vi "Test_CaseHandler.vi"(4 "data":string, 5 "action":string) -> (0 "error out":errorcluster, 1 "response":string)   [LabVIEW 2009]
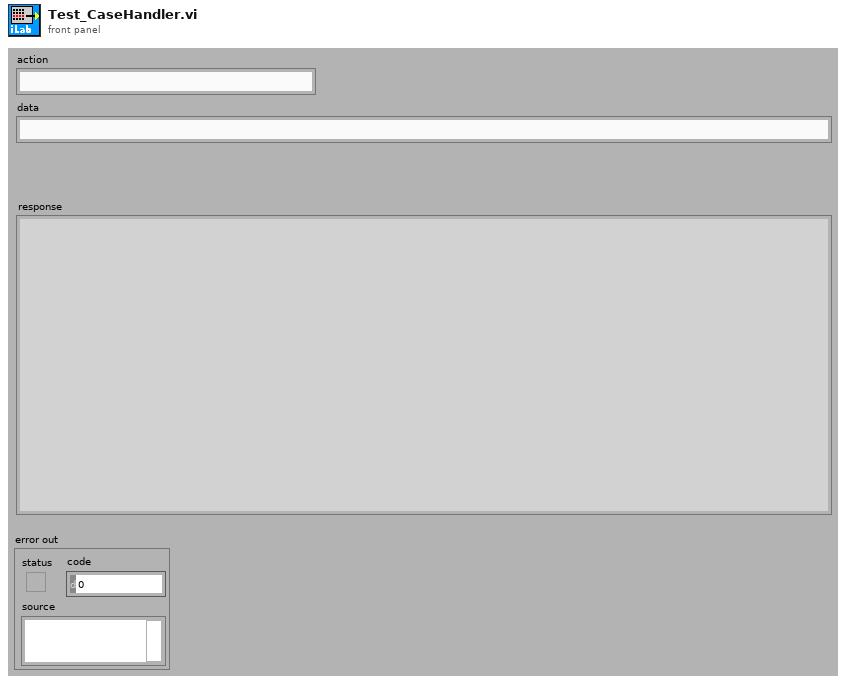
[diagram p1: front panel]
types:
  T1 = typedef "LVRemotePanelConnectionsTypeDef.ctl" = cluster{"VI Name":string, "Remote":string, "UserName":string, "Port":i32, "Status":enum32{"Viewing", "Waiting For Control", "Controlling"}, "Create Time":timestamp, "Status Time":timestamp, "Control End Time":timestamp}[]
  T2 = cluster{"VI Name":string, "Remote":string, "UserName":string, "Port":i32, "Status":enum32{"Viewing", "Waiting For Control", "Controlling"}, "Create Time":timestamp, "Status Time":timestamp, "Control End Time":timestamp}
  T3 = cluster{"Name":string, "Path":path, "Type String":string, "Display Name":string, "Type":string}
  T4 = enum32{"Bad", "Idle", "Run top level", "Running"}
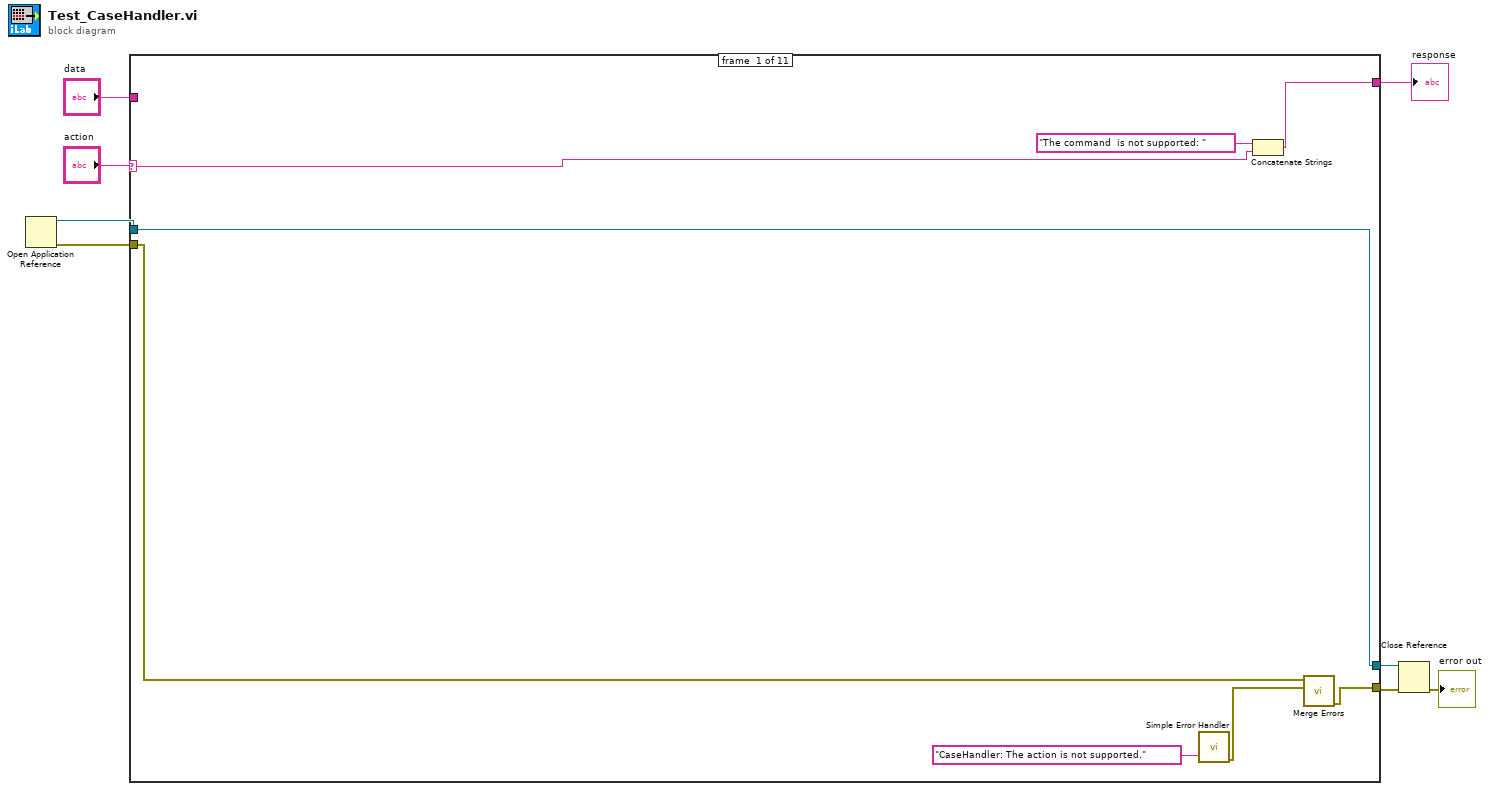
[diagram p0: block diagram]
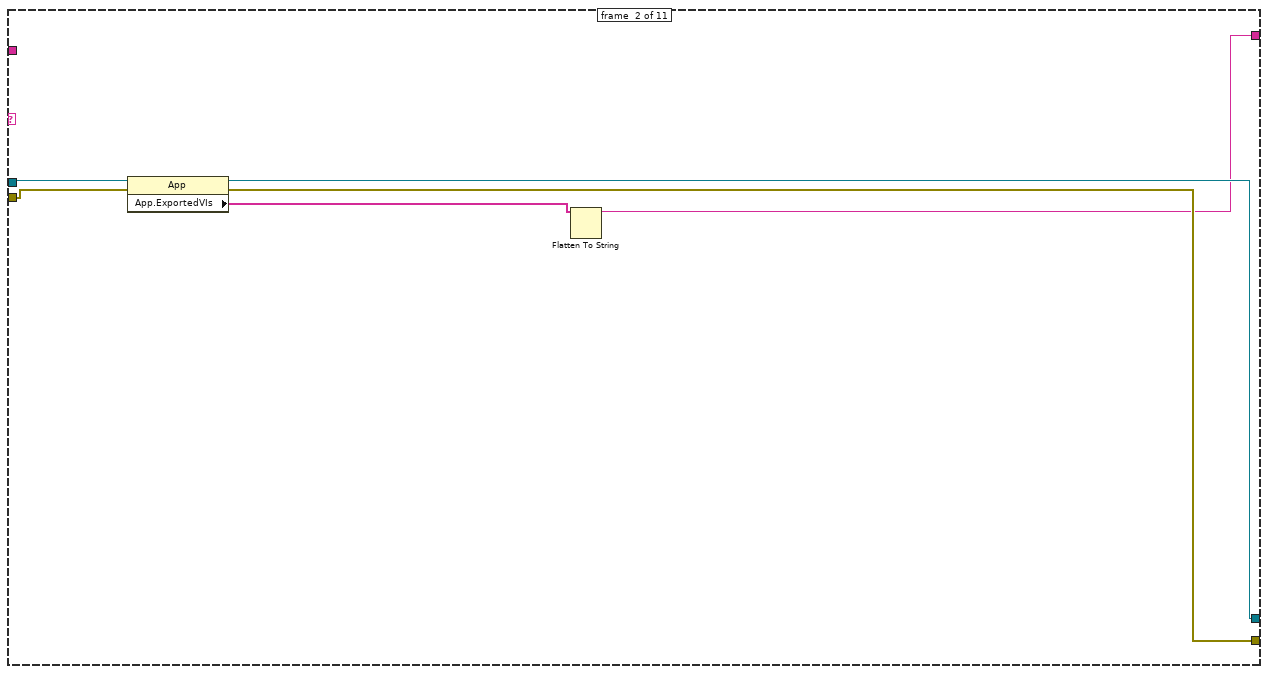
[diagram p2: hidden frame]
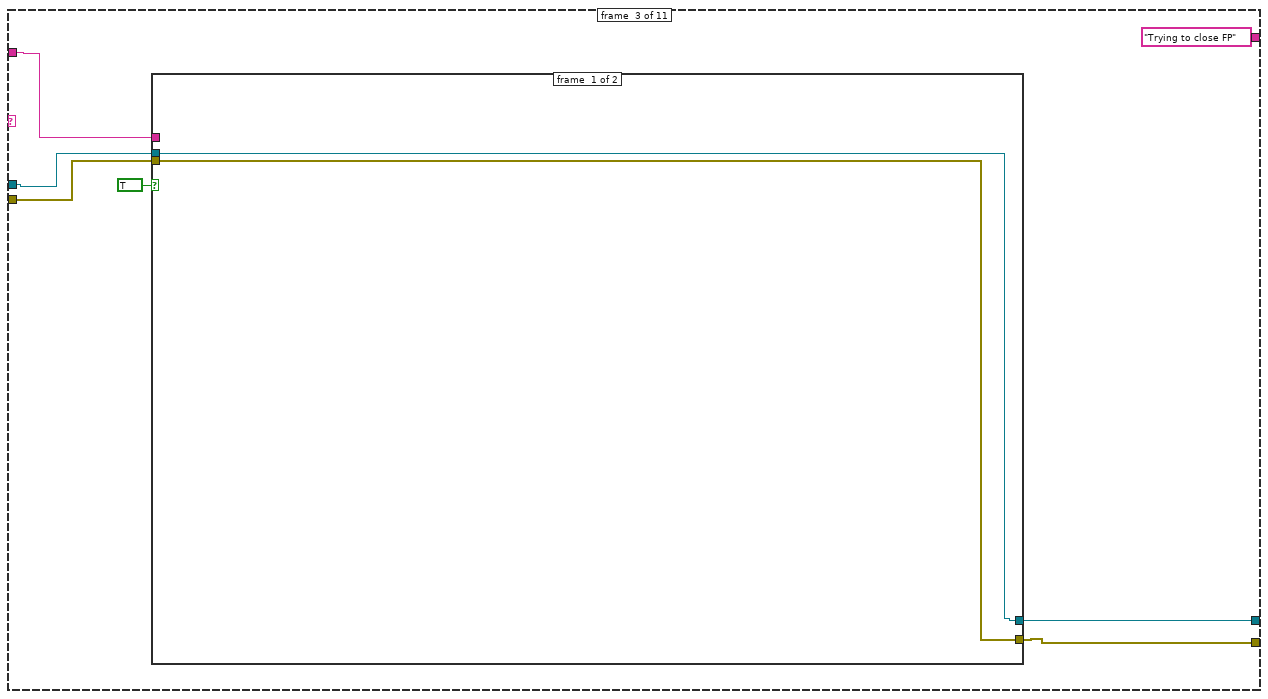
[diagram p3: hidden frame]
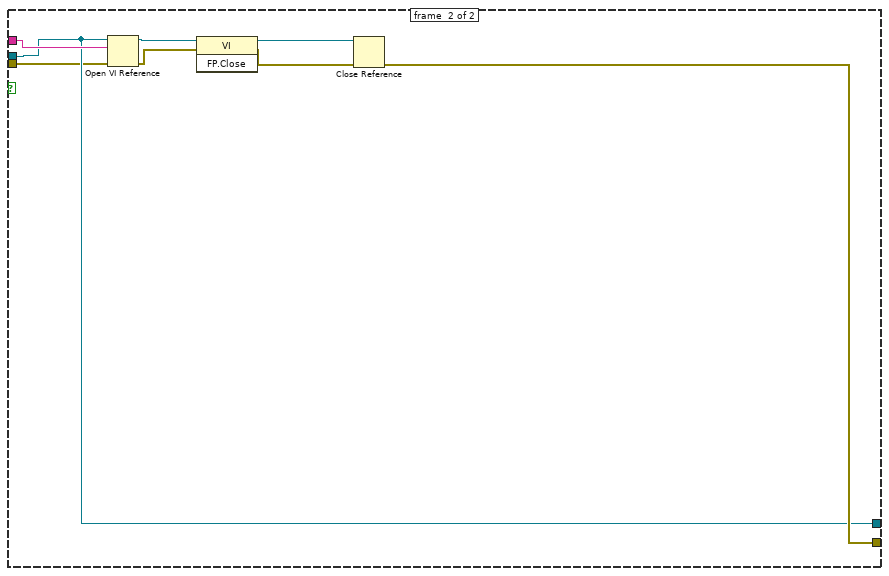
[diagram p4: hidden frame]
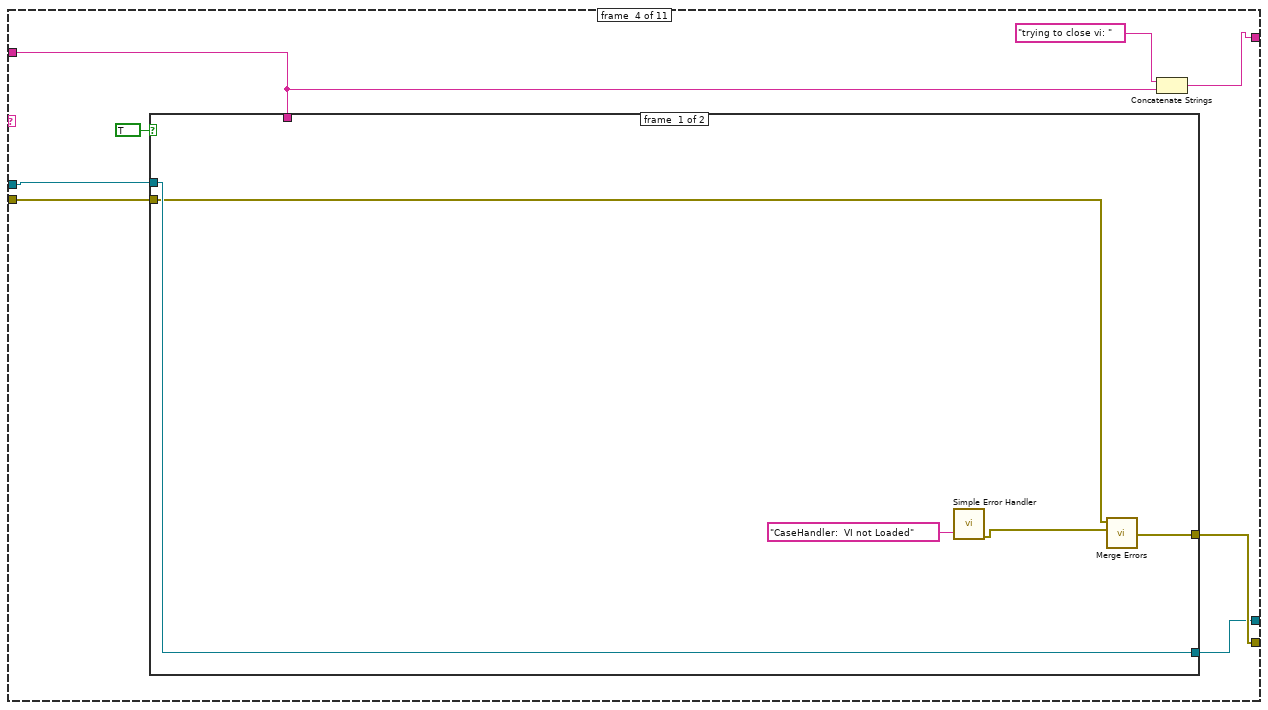
[diagram p5: hidden frame]
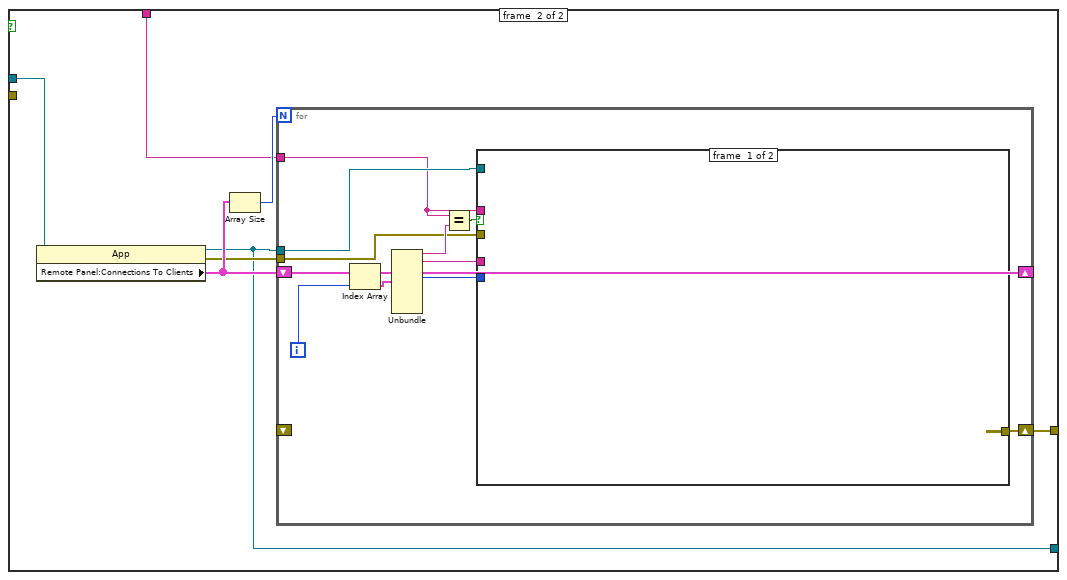
[diagram p6: hidden frame]
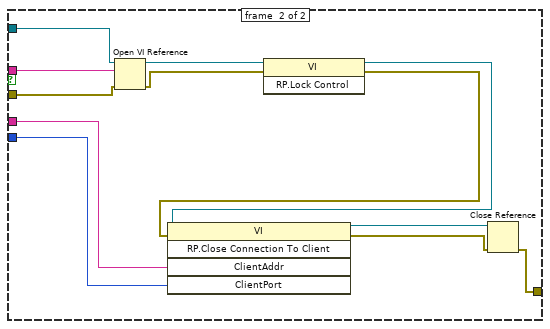
[diagram p7: hidden frame]
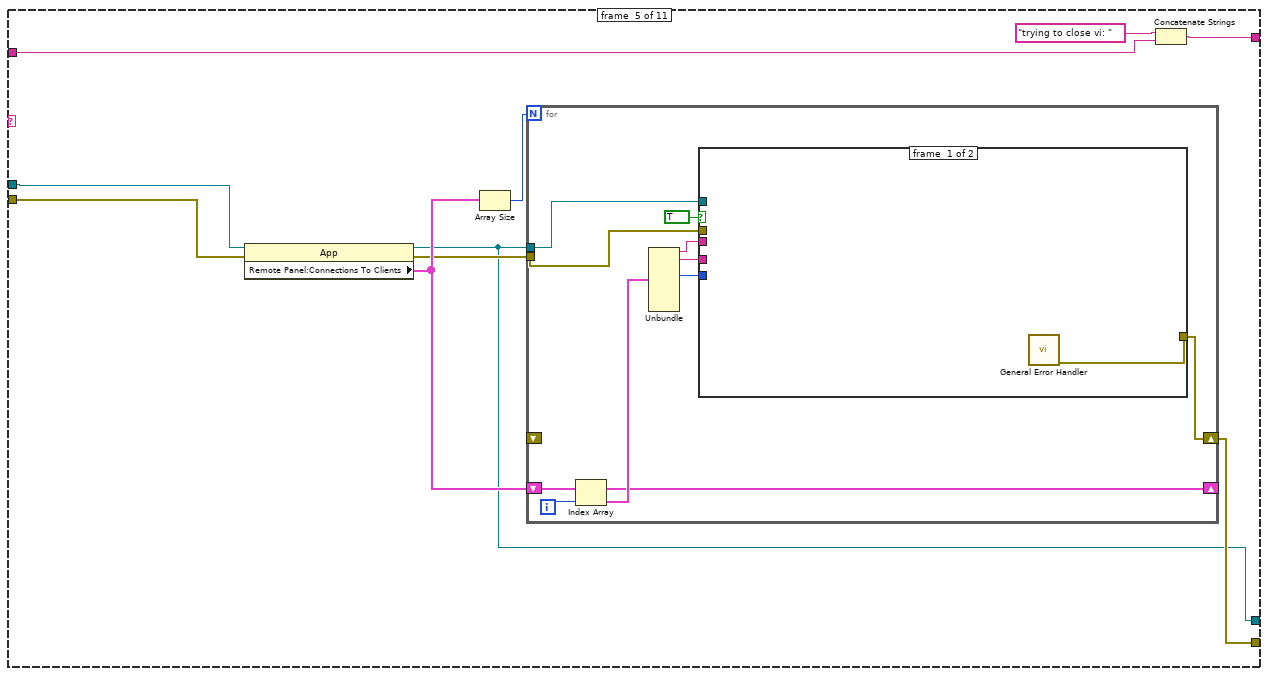
[diagram p8: hidden frame]
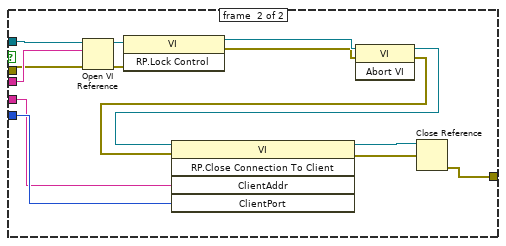
[diagram p9: hidden frame]
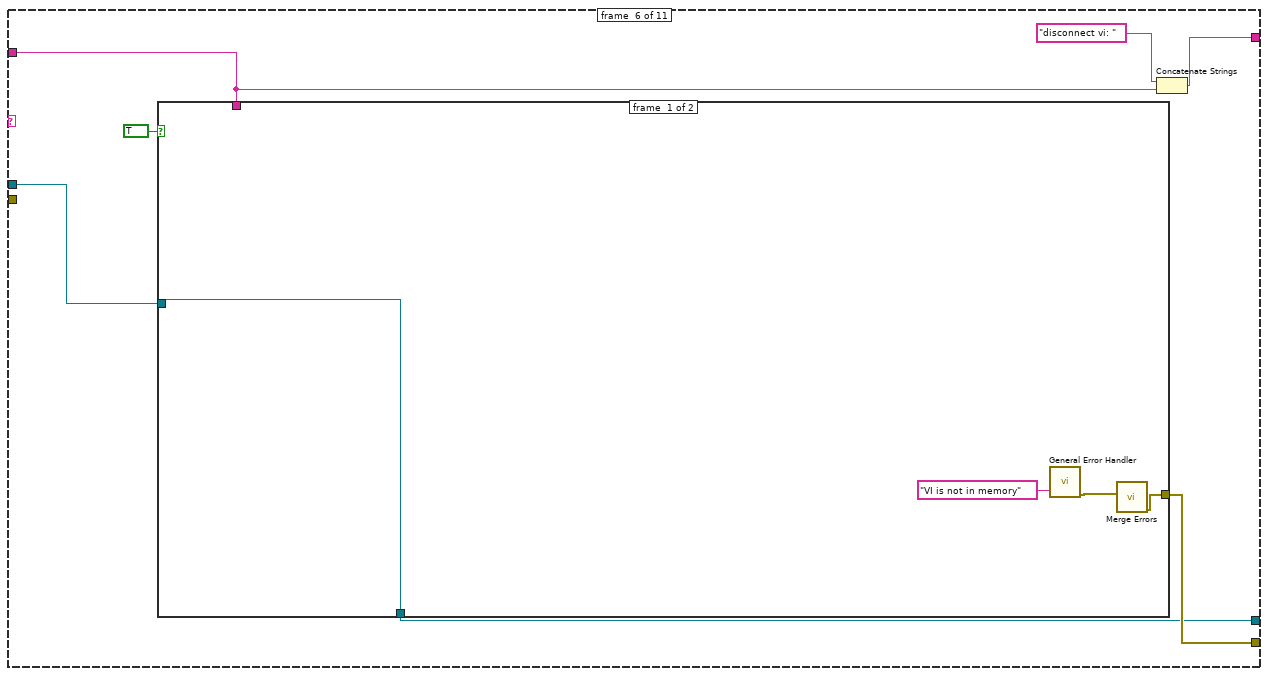
[diagram p10: hidden frame]
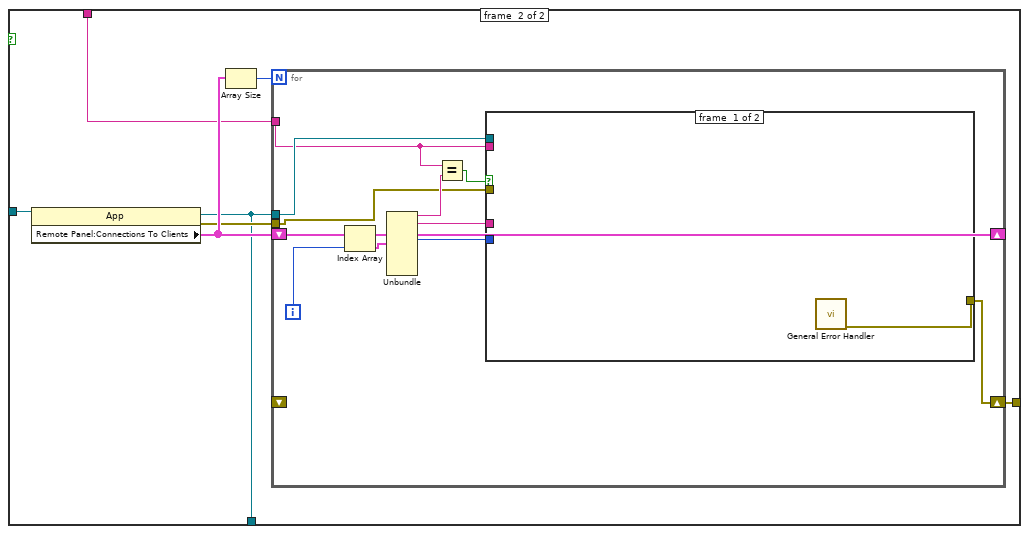
[diagram p11: hidden frame]
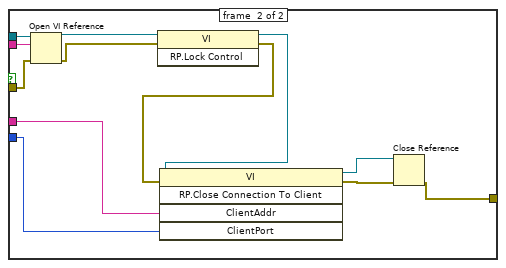
[diagram p12: hidden frame]
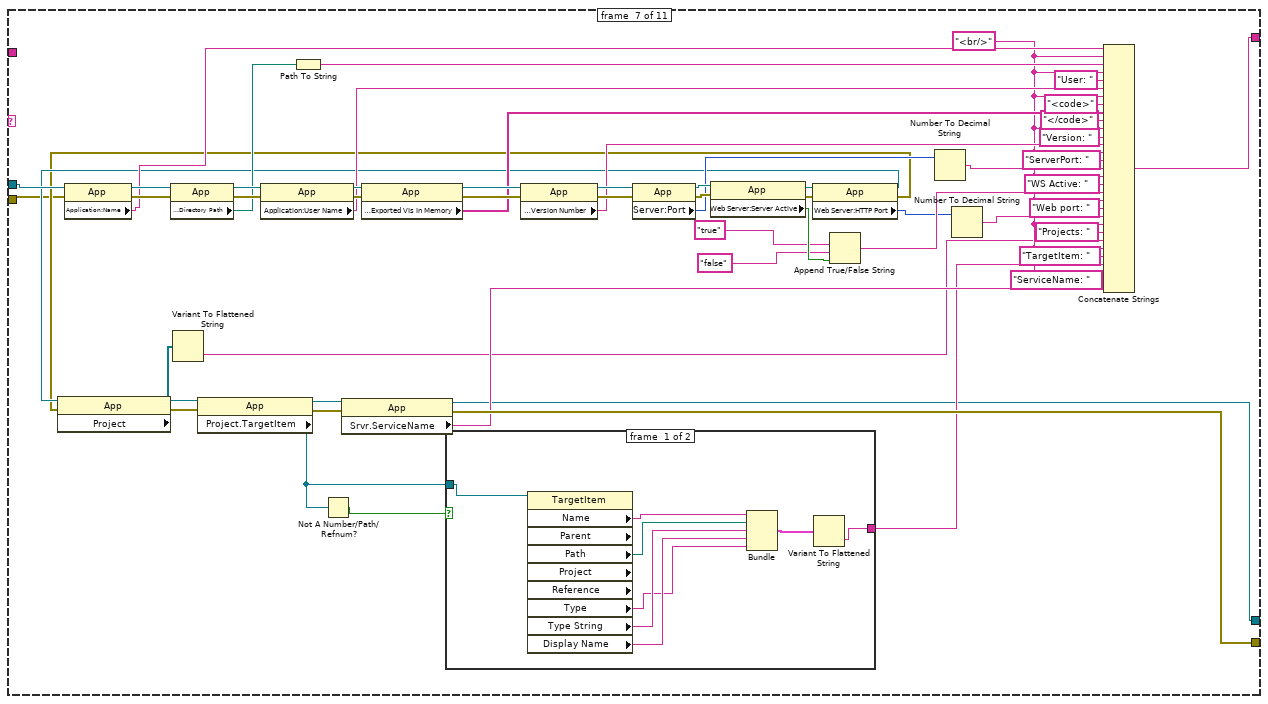
[diagram p13: hidden frame]
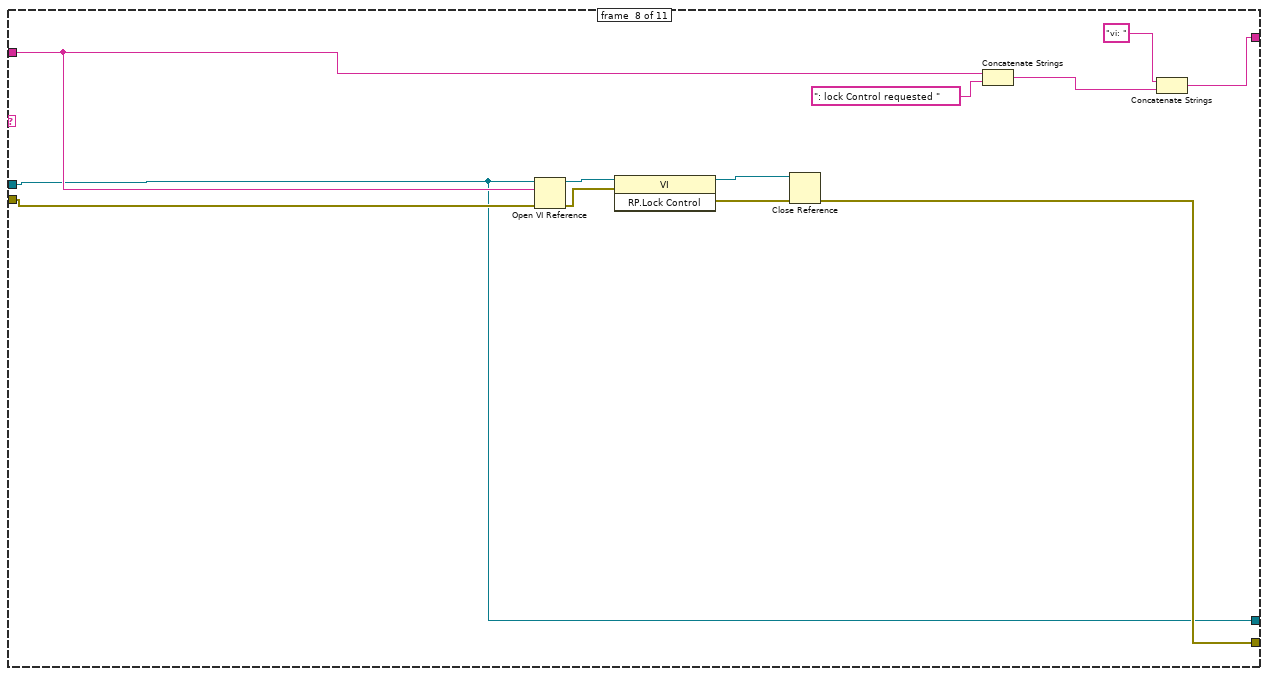
[diagram p15: hidden frame]
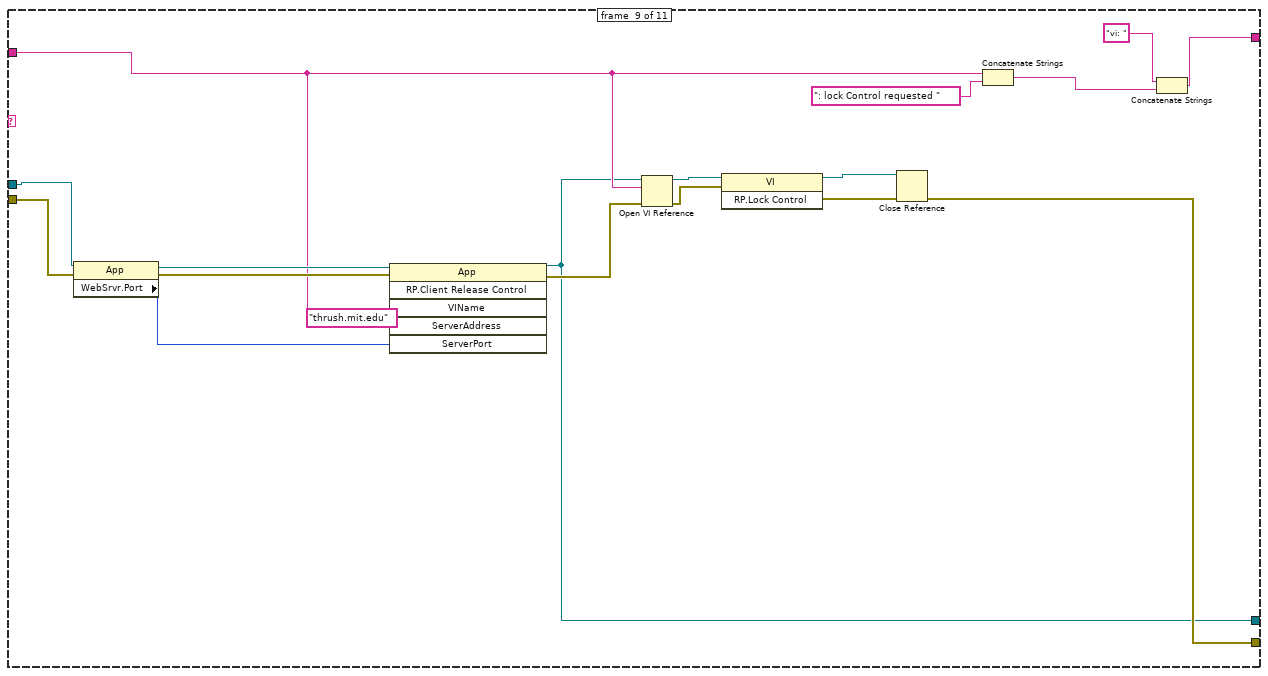
[diagram p16: hidden frame]
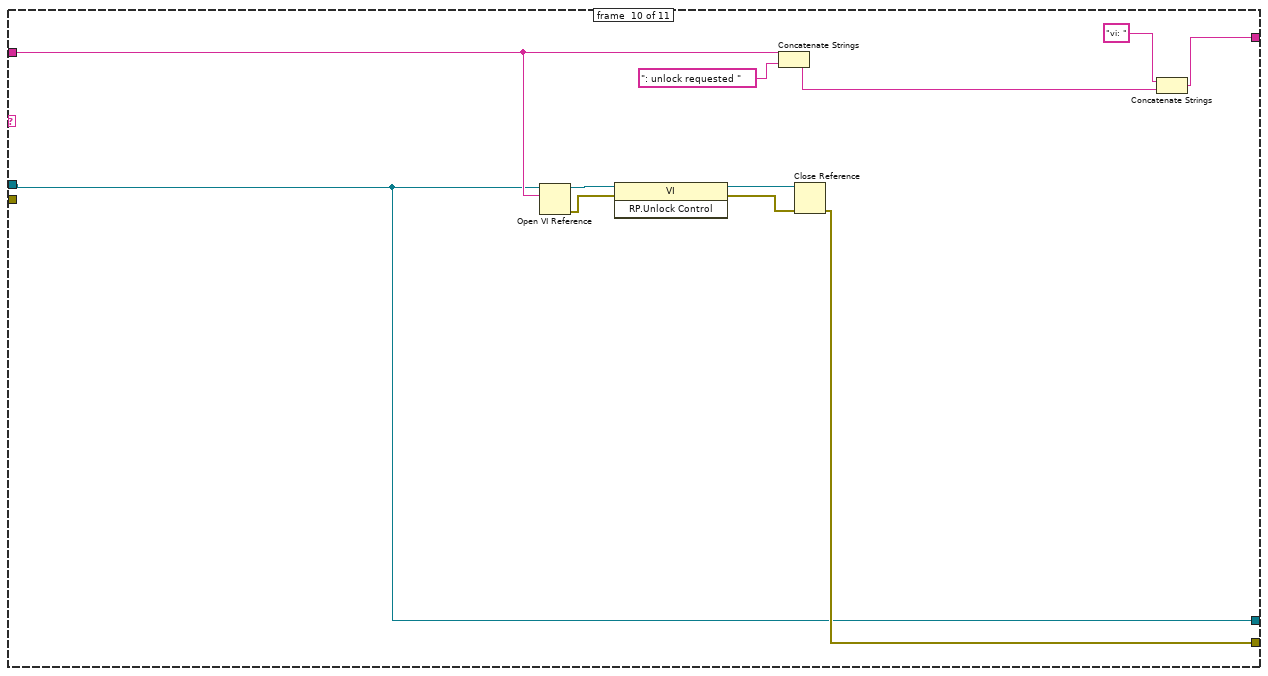
[diagram p17: hidden frame]
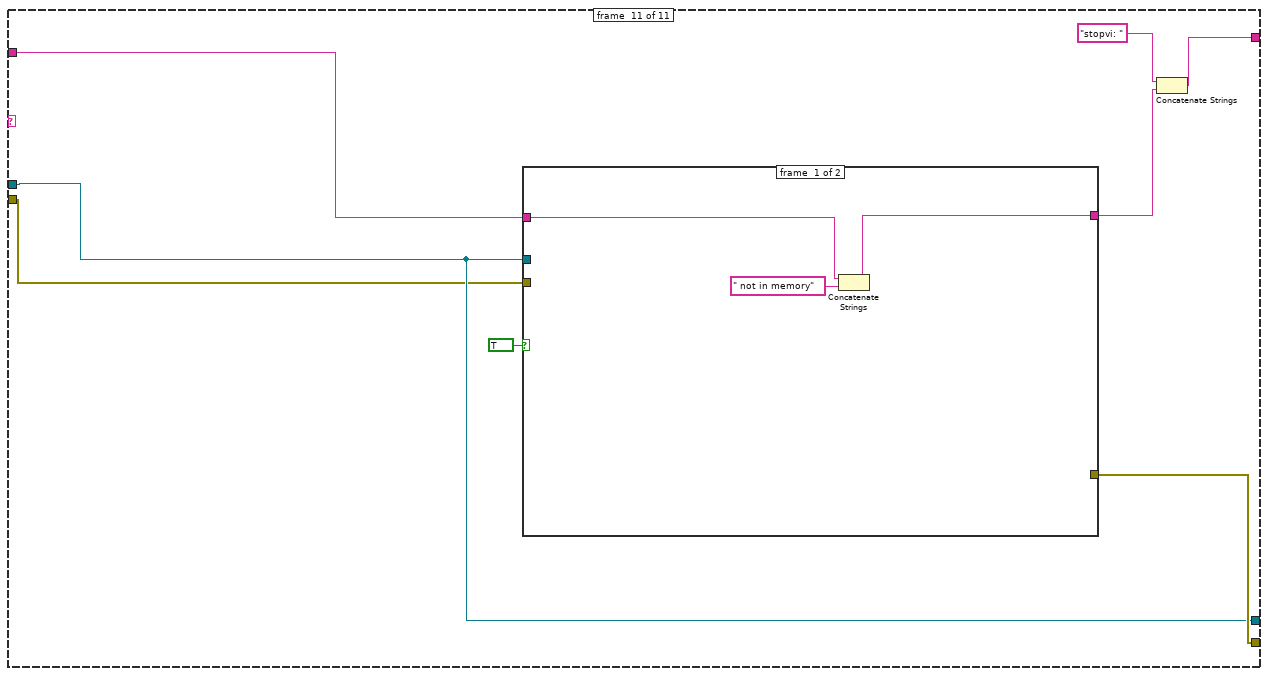
[diagram p18: hidden frame]
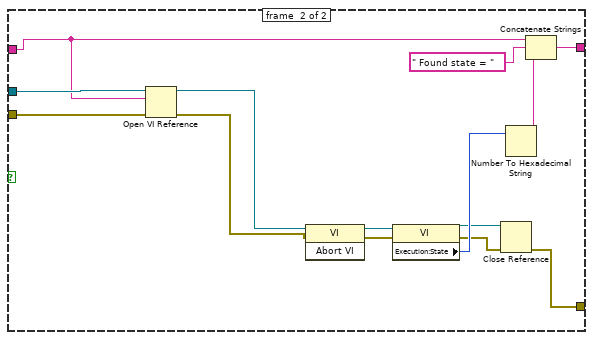
[diagram p19: hidden frame]
diagram:
  n1 = Open Application Reference() -> (0:w3:errorcluster, 3:w6:refnum<vi>)  [unwired: 1 in, 3 out]
  n2 = case shown="\"appstatus\"" "action" {
    selector: "action" -> [w15 _ _ _ _ _ _ _ _ _ _]
    tunnel: "data" -> [_ _ w29 w45 w89 w122 _ w227 w239 w256 w269]
    tunnel: [w9 w17 "Trying to close FP" ("data") w40 w83 w118 w160 w224 w236 w254 w265] -> w1
    tunnel: [w13 w19 w27 w46 w88 w123 w173 w228 w246 w257 w270] -> w5
    tunnel: w6 -> [w11 w22 w28 w44 w87 w121 w215 w225 w243 w255 w267]
    tunnel: [w11 w20 w24 w42 w84 w119 w161 w225 w237 w255 w267] -> w4
    tunnel: w3 -> [w10 w21 w25 w41 w86 _ w162 w226 w238 _ w266]
    frame #0 {
      (unwired) "The" ("message")
      n3 = call <vilib>:"Simple Error Handler.vi"("error source (\" \")"="CaseHandler: The action is not supported." ("error source (\" \")")) -> ("error out"=w12:errorcluster)  [unwired: 2 in, 6 out]
      n4 = Concatenate Strings("The command  is not supported: " ("string"), w15) -> (w9:string)
      n5 = call <vilib>:"Merge Errors.vi"("error in 2 (no error)"=w12, "error in 1 (no error)"=w10) -> ("error out"=w13:errorcluster)  [unwired: 2 in, 3 out]
    }
    frame #1 {
      n6 = property class="App"(reference=w22, error in=w21) -> (reference out=w20:refnum<vi>, error out=w19:errorcluster, "App.ExportedVIs"=w18:string[])
      n7 = Flatten To String(anything=w18) -> (data string=w17:string)  [unwired: 1 in, 4 out]
    }
    frame #2 {
      n8 = case shown="False" TRUE {
        tunnel: w29 -> [_ w34]
        tunnel: w28 -> [w31 w33]
        tunnel: [w30 w35] -> w27
        tunnel: [w31 w33] -> w24
        tunnel: w25 -> [w30 w32]
        frame #0 {
        }
        frame #1 {
          n9 = Open VI Reference(application reference (local)=w33, vi path=w34, error in (no error)=w32) -> (vi reference=w39:refnum<vi>, error out=w38:errorcluster)  [unwired: 3 out]
          n10 = invoke class="VI" method="FP.Close"(reference=w39, error in=w38) -> (reference out=w37:refnum<vi>, error out=w36:errorcluster)  [unwired: 1 in, 1 out]
          n11 = Close Reference(reference=w37, error in (no error)=w36) -> (error out=w35:errorcluster)
        }
      }
    }
    frame #3 {
      n12 = case shown="False" TRUE {
        tunnel: [w48 w57] -> w46
        tunnel: w45 -> [_ w56]
        tunnel: w44 -> [w51 w55]
        tunnel: [w51 w53] -> w42
        tunnel: w41 -> [w50 _]
        frame #0 {
          n13 = call <vilib>:"Simple Error Handler.vi"("error source (\" \")"="CaseHandler:  VI not Loaded" ("error source (\" \")")) -> ("error out"=w49:errorcluster)  [unwired: 2 in, 6 out]
          n14 = call <vilib>:"Merge Errors.vi"("error in 2 (no error)"=w49, "error in 1 (no error)"=w50) -> ("error out"=w48:errorcluster)  [unwired: 2 in, 3 out]
        }
        frame #1 {
          n15 = property class="App"(reference=w55) -> (reference out=w53:refnum<vi>, error out=w54:errorcluster, "Remote Panel:Connections To Clients"=w58:T1)  [unwired: 1 in]
          n16 = Array Size(array=w58) -> (size(s)=w59:i32)
          n17 = for {
            N: w59 -> [_]
            shift-right: [w63] -> _
            shift-left: w58 -> [w63]
            tunnel: w56 -> [w61]
            shift-right: [w65] -> w57
            shift-left: _ -> [_]
            tunnel: w53 -> [w62]
            tunnel: w54 -> [w60]
            i -> [w70]
            n18 = Index Array(array=w63, index=w70) -> (element=w69:T2)
            n19 = Unbundle(w69) -> ("VI Name"=w64:string, "Remote"=w66:string, "Port"=w67:i32)  [unwired: 5 out]
            n20 = Equal?(x=w61, y=w64) -> (x = y?=w68:bool)
            n21 = case shown="True" w68 {
              tunnel: w67 -> [_ w82]
              tunnel: w66 -> [_ w81]
              tunnel: [_ w80] -> w65
              tunnel: w62 -> [_ w71]
              tunnel: w61 -> [_ w77]
              tunnel: w60 -> [_ w74]
              frame #0 {
              }
              frame #1 {
                n22 = Open VI Reference(application reference (local)=w71, vi path=w77, error in (no error)=w74) -> (vi reference=w73:refnum<vi>, error out=w72:errorcluster)  [unwired: 3 out]
                n23 = invoke class="VI" method="RP.Lock Control"(reference=w73, error in=w72) -> (reference out=w76:refnum<vi>, error out=w75:errorcluster)  [unwired: 1 in, 1 out]
                n24 = invoke class="VI" method="RP.Close Connection To Client"(reference=w76, error in=w75, "ClientAddr"=w81, "ClientPort"=w82) -> (reference out=w78:refnum<vi>, error out=w79:errorcluster)  [unwired: 1 in, 3 out]
                n25 = Close Reference(reference=w78, error in (no error)=w79) -> (error out=w80:errorcluster)
              }
            }
          }
        }
      }
      n26 = Concatenate Strings("trying to close vi: " ("data"), w45) -> (w40:string)
    }
    frame #4 {
      n27 = property class="App"(reference=w87, error in=w86) -> (reference out=w84:refnum<vi>, error out=w85:errorcluster, "Remote Panel:Connections To Clients"=w91:T1)
      n28 = Array Size(array=w91) -> (size(s)=w92:i32)
      n29 = for {
        N: w92 -> [_]
        shift-right: [w96] -> _
        shift-left: w91 -> [w96]
        shift-right: [w98] -> w88
        shift-left: _ -> [_]
        tunnel: w84 -> [w95]
        tunnel: w85 -> [w93]
        i -> [w102]
        n30 = Index Array(array=w96, index=w102) -> (element=w101:T2)
        n31 = Unbundle(w101) -> ("VI Name"=w97:string, "Remote"=w99:string, "Port"=w100:i32)  [unwired: 5 out]
        n32 = case shown="True" TRUE {
          tunnel: w100 -> [_ w117]
          tunnel: w99 -> [_ w116]
          tunnel: [w103 w115] -> w98
          tunnel: w97 -> [_ w114]
          tunnel: w95 -> [_ w105]
          tunnel: w93 -> [_ w104]
          frame #0 {
            n33 = call <vilib>:"General Error Handler.vi"() -> ("error out"=w103:errorcluster)  [unwired: 2 in, 13 out]
          }
          frame #1 {
            n34 = Open VI Reference(application reference (local)=w105, vi path=w114, error in (no error)=w104) -> (vi reference=w109:refnum<vi>, error out=w108:errorcluster)  [unwired: 1 in, 2 out]
            n35 = invoke class="VI" method="RP.Lock Control"(reference=w109, error in=w108) -> (reference out=w107:refnum<vi>, error out=w106:errorcluster)  [unwired: 1 in, 1 out]
            n36 = invoke class="VI" method="Abort VI"(reference=w107, error in=w106) -> (reference out=w110:refnum<vi>, error out=w111:errorcluster)  [unwired: 1 in, 1 out]
            n37 = invoke class="VI" method="RP.Close Connection To Client"(reference=w110, error in=w111, "ClientAddr"=w116, "ClientPort"=w117) -> (reference out=w113:refnum<vi>, error out=w112:errorcluster)  [unwired: 1 in, 3 out]
            n38 = Close Reference(reference=w113, error in (no error)=w112) -> (error out=w115:errorcluster)
          }
        }
      }
      n39 = Concatenate Strings("trying to close vi: " ("data"), w89) -> (w83:string)
    }
    frame #5 {
      n40 = case shown="False" TRUE {
        tunnel: [w125 w133] -> w123
        tunnel: w122 -> [_ w132]
        tunnel: w121 -> [w127 w131]
        tunnel: [w127 w129] -> w119
        frame #0 {
          n41 = call <vilib>:"General Error Handler.vi"("[error source] (\" \")"="VI is not in memory" ("[error source] (\" \")")) -> ("error out"=w126:errorcluster)  [unwired: 2 in, 12 out]
          n42 = call <vilib>:"Merge Errors.vi"("error in 2 (no error)"=w126) -> ("error out"=w125:errorcluster)  [unwired: 3 in, 3 out]
        }
        frame #1 {
          n43 = property class="App"(reference=w131) -> (reference out=w129:refnum<vi>, error out=w130:errorcluster, "Remote Panel:Connections To Clients"=w134:T1)  [unwired: 1 in]
          n44 = Array Size(array=w134) -> (size(s)=w135:i32)
          n45 = for {
            N: w135 -> [_]
            shift-right: [w139] -> _
            shift-left: w134 -> [w139]
            tunnel: w132 -> [w136]
            shift-right: [w141] -> w133
            shift-left: _ -> [_]
            tunnel: w129 -> [w138]
            tunnel: w130 -> [w137]
            i -> [w146]
            n46 = Index Array(array=w139, index=w146) -> (element=w145:T2)
            n47 = Unbundle(w145) -> ("VI Name"=w140:string, "Remote"=w142:string, "Port"=w143:i32)  [unwired: 5 out]
            n48 = Equal?(x=w136, y=w140) -> (x = y?=w144:bool)
            n49 = case shown="True" w144 {
              tunnel: w143 -> [_ w159]
              tunnel: w142 -> [_ w158]
              tunnel: [w147 w150] -> w141
              tunnel: w138 -> [_ w153]
              tunnel: w137 -> [_ w149]
              tunnel: w136 -> [_ w148]
              frame #0 {
                n50 = call <vilib>:"General Error Handler.vi"() -> ("error out"=w147:errorcluster)  [unwired: 2 in, 13 out]
              }
              frame #1 {
                n51 = Open VI Reference(application reference (local)=w153, vi path=w148, error in (no error)=w149) -> (vi reference=w157:refnum<vi>, error out=w154:errorcluster)  [unwired: 3 out]
                n52 = invoke class="VI" method="RP.Lock Control"(reference=w157, error in=w154) -> (reference out=w156:refnum<vi>, error out=w155:errorcluster)  [unwired: 1 in, 1 out]
                n53 = invoke class="VI" method="RP.Close Connection To Client"(reference=w156, error in=w155, "ClientAddr"=w158, "ClientPort"=w159) -> (reference out=w151:refnum<vi>, error out=w152:errorcluster)  [unwired: 1 in, 3 out]
                n54 = Close Reference(reference=w151, error in (no error)=w152) -> (error out=w150:errorcluster)
              }
            }
          }
        }
      }
      n55 = Concatenate Strings("disconnect vi: " ("data"), w122) -> (w118:string)
    }
    frame #6 {
      w171 = "<br/>" ("string")
      n56 = property class="App"(reference=w215, error in=w162) -> (reference out=w214:refnum<vi>, error out=w209:errorcluster, "Application:Name"=w200:string)
      n57 = property class="App"(reference=w214, error in=w209) -> (reference out=w213:refnum<vi>, error out=w208:errorcluster, "Application:Directory Path"=w198:path)
      n58 = property class="App"(reference=w213, error in=w208) -> (reference out=w212:refnum<vi>, error out=w207:errorcluster, "Application:User Name"=w196:string)
      n59 = Path To String(path=w198) -> (string=w199:string)
      n60 = property class="App"(reference=w212, error in=w207) -> (reference out=w211:refnum<vi>, error out=w206:errorcluster, "Application:Exported VIs In Memory"=w194:string[])
      n61 = property class="App"(reference=w211, error in=w206) -> (reference out=w210:refnum<vi>, error out=w205:errorcluster, "Application:Version Number"=w191:string)
      n62 = property class="App"(reference=w210, error in=w205) -> (reference out=w201:refnum<vi>, error out=w202:errorcluster, "Server:Port"=w188:u32)
      n63 = property class="App"(reference=w201, error in=w202) -> (reference out=w204:refnum<vi>, error out=w203:errorcluster, "Web Server:Server Active"=w186:bool)
      n64 = property class="App"(reference=w204, error in=w203) -> (reference out=w179:refnum<vi>, error out=w176:errorcluster, "Web Server:HTTP Port"=w181:u16)
      n65 = property class="App"(reference=w179, error in=w176) -> (reference out=w178:refnum<vi>, error out=w175:errorcluster, "Project"=w167:refnum<vi>[])
      n66 = Variant To Flattened String(Variant=w167) -> (data string=w166:string)  [unwired: 1 out]
      n67 = property class="App"(reference=w178, error in=w175) -> (reference out=w177:refnum<vi>, error out=w174:errorcluster, "Project.TargetItem"=w163:refnum<vi>)
      n68 = Not A Number/Path/Refnum?(number/path/refnum=w163) -> (NaN/Path/Refnum?=w164:bool)
      n69 = property class="App"(reference=w177, error in=w174) -> (reference out=w161:refnum<vi>, error out=w173:errorcluster, "Srvr.ServiceName"=w168:string)
      n70 = case shown="True" w164 {
        tunnel: [w217 _] -> w165
        tunnel: w163 -> [w216 _]
        frame #0 {
          n71 = property class="TargetItem" props=["Name", "Parent", "Path", "Project", "Reference", "Type", "Type String", "Display Name"](reference=w216) -> ("Name"=w223:string, "Path"=w222:path, "Type"=w219:string, "Type String"=w221:string, "Display Name"=w220:string)  [unwired: 1 in, 5 out]
          n72 = Bundle("Name"=w223, "Path"=w222, "Type String"=w221, "Display Name"=w220, "Type"=w219) -> (w218:T3)  [unwired: 1 out]
          n73 = Variant To Flattened String(Variant=w218) -> (data string=w217:string)  [unwired: 1 out]
        }
        frame #1 {
        }
      }
      n74 = Append True/False String(1:w186, 2:"false" ("false string"), 3:"true" ("true string")) -> (0:w185:string)  [unwired: 1 out]
      n75 = Number To Decimal String(number=w188) -> (decimal integer string=w189:string)  [unwired: 1 out]
      n76 = Number To Decimal String(number=w181) -> (decimal integer string=w180:string)  [unwired: 1 out]
      n77 = Concatenate Strings(w200, w171, w199, w171, "User: " ("string"), w196, w171, "<code>" ("string"), w194, "</code>" ("string"), w171, "Version: " ("string"), w191, w171, "ServerPort: " ("string"), w189, w171, "WS Active: " ("string"), w185, w171, "Web port: " ("string"), w180, w171, "Projects: " ("string"), w166, w171, "TargetItem: " ("string"), w165, w171, "ServiceName: " ("string"), w168) -> (w160:string)
    }
    frame #7 {
      n78 = Open VI Reference(application reference (local)=w225, vi path=w227, error in (no error)=w226) -> (vi reference=w234:refnum<vi>, error out=w233:errorcluster)  [unwired: 3 out]
      n79 = invoke class="VI" method="RP.Lock Control"(reference=w234, error in=w233) -> (reference out=w231:refnum<vi>, error out=w230:errorcluster)  [unwired: 1 in, 1 out]
      n80 = Close Reference(reference=w231, error in (no error)=w230) -> (error out=w228:errorcluster)
      n81 = Concatenate Strings(w227, ": lock Control requested " ("string")) -> (w229:string)
      n82 = Concatenate Strings("vi: " ("data"), w229) -> (w224:string)
    }
    frame #8 {
      n83 = property class="App"(reference=w243, error in=w238) -> (reference out=w242:refnum<vi>, error out=w240:errorcluster, "WebSrvr.Port"=w245:u16)
      n84 = invoke class="App" method="RP.Client Release Control"(reference=w242, error in=w240, "VIName"=w239, "ServerAddress"="thrush.mit.edu" ("Server Address"), "ServerPort"=w245) -> (reference out=w237:refnum<vi>, error out=w241:errorcluster)  [unwired: 1 in, 4 out]
      n85 = Open VI Reference(application reference (local)=w237, vi path=w239, error in (no error)=w241) -> (vi reference=w252:refnum<vi>, error out=w251:errorcluster)  [unwired: 3 out]
      n86 = invoke class="VI" method="RP.Lock Control"(reference=w252, error in=w251) -> (reference out=w249:refnum<vi>, error out=w248:errorcluster)  [unwired: 1 in, 1 out]
      n87 = Close Reference(reference=w249, error in (no error)=w248) -> (error out=w246:errorcluster)
      n88 = Concatenate Strings(w239, ": lock Control requested " ("string")) -> (w247:string)
      n89 = Concatenate Strings("vi: " ("data"), w247) -> (w236:string)
    }
    frame #9 {
      n90 = Open VI Reference(application reference (local)=w255, vi path=w256) -> (vi reference=w263:refnum<vi>, error out=w262:errorcluster)  [unwired: 1 in, 3 out]
      n91 = invoke class="VI" method="RP.Unlock Control"(reference=w263, error in=w262) -> (reference out=w260:refnum<vi>, error out=w259:errorcluster)  [unwired: 1 in, 1 out]
      n92 = Concatenate Strings(w256, ": unlock requested " ("string")) -> (w258:string)
      n93 = Close Reference(reference=w260, error in (no error)=w259) -> (error out=w257:errorcluster)
      n94 = Concatenate Strings("vi: " ("data"), w258) -> (w254:string)
    }
    frame #10 {
      n95 = case shown="True" TRUE {
        tunnel: w269 -> [w275 w277]
        tunnel: [_ w280] -> w270
        tunnel: [w274 w287] -> w271
        tunnel: w267 -> [_ w283]
        tunnel: w266 -> [_ w276]
        frame #0 {
          n96 = Concatenate Strings(w275, " not in memory" ("string")) -> (w274:string)
        }
        frame #1 {
          n97 = Open VI Reference(application reference (local)=w283, vi path=w277, error in (no error)=w276) -> (vi reference=w279:refnum<vi>, error out=w278:errorcluster)  [unwired: 1 in, 2 out]
          n98 = invoke class="VI" method="Abort VI"(reference=w279, error in=w278) -> (reference out=w285:refnum<vi>, error out=w284:errorcluster)  [unwired: 1 in, 1 out]
          n99 = property class="VI"(reference=w285, error in=w284) -> (reference out=w282:refnum<vi>, error out=w281:errorcluster, "Execution:State"=w289:T4)
          n100 = Close Reference(reference=w282, error in (no error)=w281) -> (error out=w280:errorcluster)
          n101 = Number To Hexadecimal String(2:w289) -> (0:w288:string)  [unwired: 1 out]
          n102 = Concatenate Strings(w277, " Found state = " ("string"), w288) -> (w287:string)
        }
      }
      n103 = Concatenate Strings("stopvi: " ("data"), w271) -> (w265:string)
    }
  }
  "response" <- w1
  n104 = Close Reference(reference=w4, error in (no error)=w5) -> (error out=→"error out":errorcluster)
